vi "Output_CSV.vi"(9 "資料Array":string[][](array[string]), 10 "檔名":string, 11 "今日存放位置":path) -> (0 "error out":errorcluster)   [LabVIEW 2019]
uses:
  <vilib>/Utility/file.llb/Write Delimited Spreadsheet (string).vi
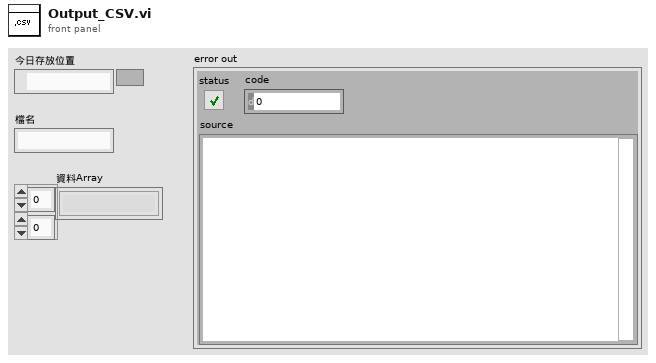
[diagram p1: front panel]
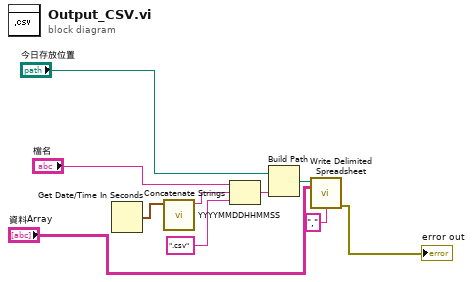
[diagram p0: block diagram]
diagram:
  n1 = Get Date/Time In Seconds() -> (seconds since 1Jan1904=w1:timestamp)
  n2 = call "YYYYMMDDHHMMSS.vi"("seconds since 1Jan1904"=w1) -> ("result string"=w3:string)  [unwired: 10 in]
  n3 = Concatenate Strings("檔名", w3, ".csv" ("string")) -> (w5:string)
  n4 = Build Path(base path="今日存放位置", name or relative path=w5) -> (appended path=w7:path)
  n5 = call-poly <vilib>:"Write Delimited Spreadsheet.vi"("file path (dialog if empty)"=w7, "2D data"="資料Array", "delimiter (\\t)"="," ("delimiter (\\t)")) -> ("error out"=→"error out":errorcluster)  [unwired: 11 in, 1 out]
